vi "Initialise State.vi"(8 "error in (no error)":errorcluster, 11 "Event_Polled Type.lvclass in":refnum<class "Event_Polled Type.lvclass">) -> (0 "error out":errorcluster, 3 "Event_Polled Type.lvclass out":refnum<class "Event_Polled Type.lvclass">)   [LabVIEW 2021, in "Event_Polled Type.lvclass"]
uses:
  Event_Polled Type.lvclass
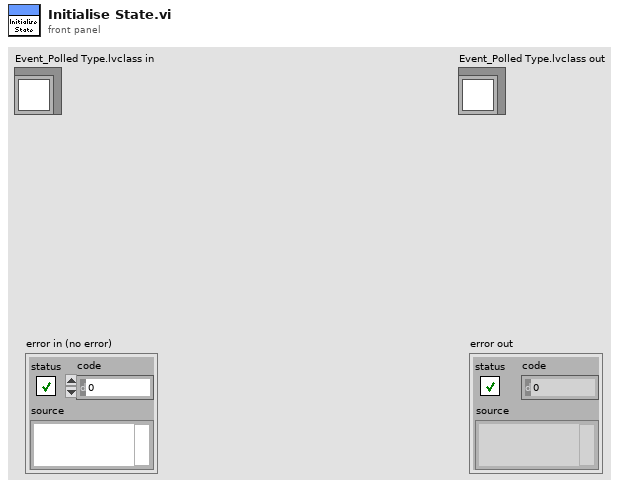
[diagram p1: front panel]
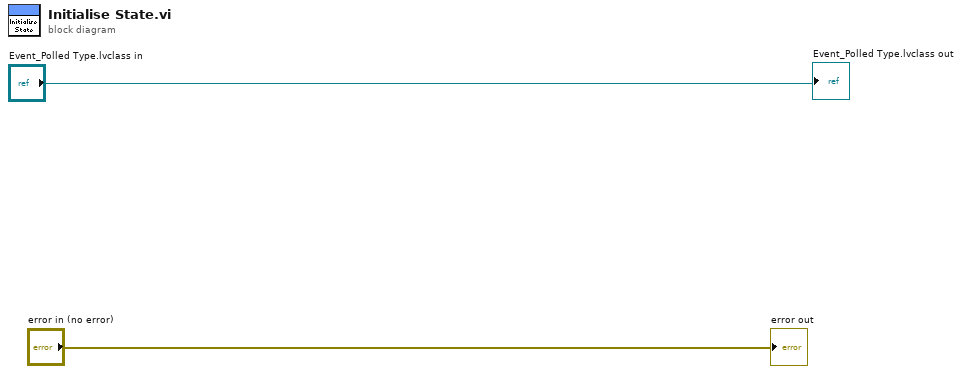
[diagram p0: block diagram]
diagram:
  "error out" <- "error in (no error)"
  "Event_Polled Type.lvclass out" <- "Event_Polled Type.lvclass in"
